vi "getQBData.vi"(8 "error in (no error)":errorcluster, 10 "path":path) -> (0 "error out":errorcluster, 2 "data":string[][](array[string]))   [LabVIEW 2012]
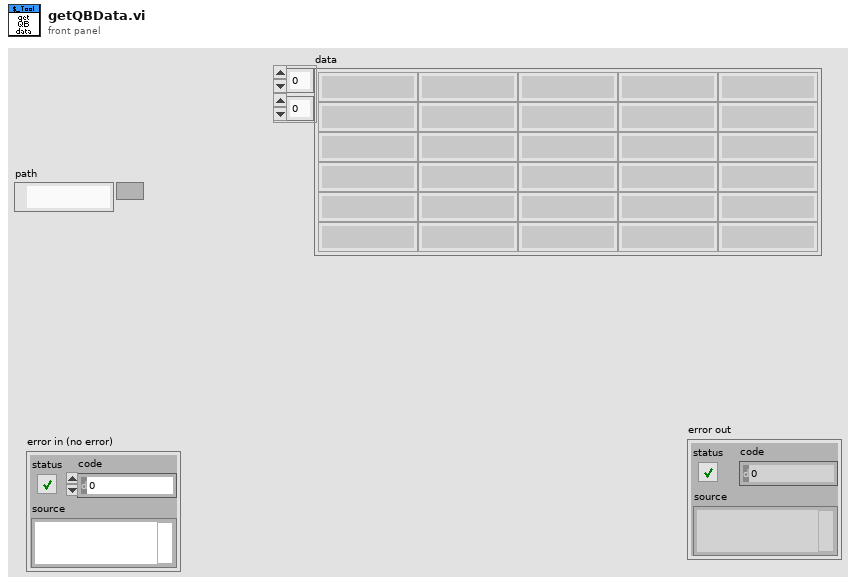
[diagram p1: front panel]
types:
  T1 = cluster{"Excel._Application":refnum<k7>, "Workbooks":refnum<k7>, "Open":refnum<k7>, "Worksheets":refnum<k7>, "Excel._Worksheet":refnum<k7>}
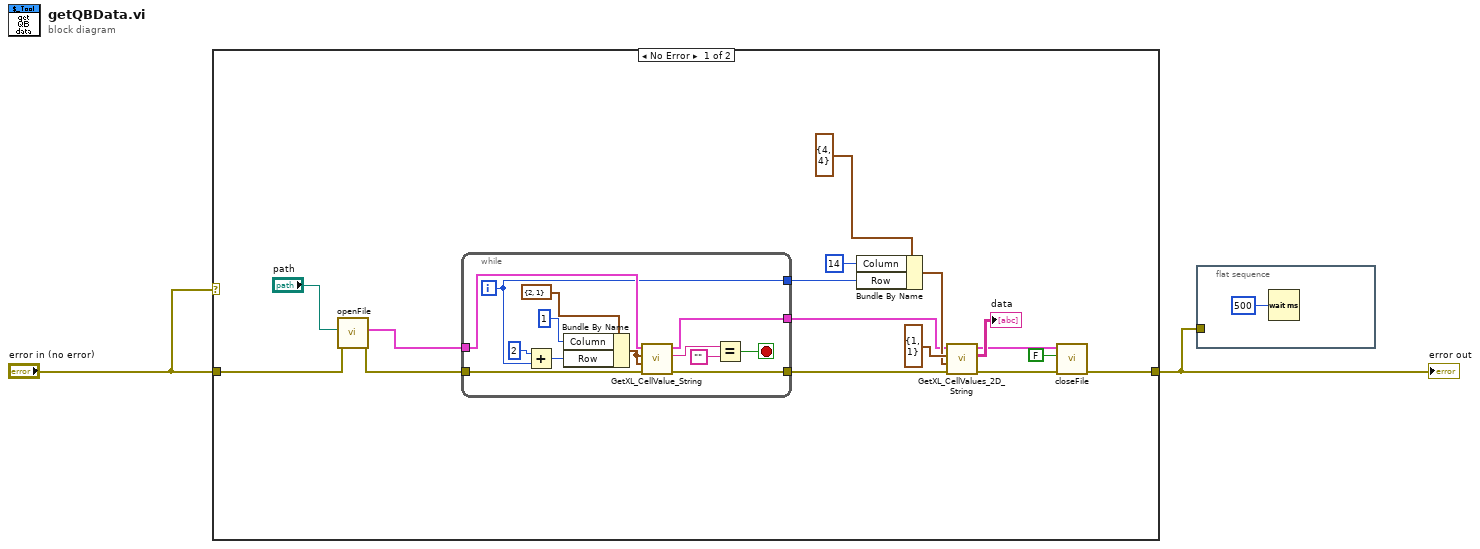
[diagram p0: block diagram]
diagram:
  n1 = case shown="No Error" "error in (no error)" {
    tunnel: "error in (no error)" -> [w8 w32]
    tunnel: [w5 w32] -> w1
    frame No Error {
      n2 = call "openFile.vi"("error in (no error)"=w8, "path"="path") -> ("error out"=w7:errorcluster, "Refnum Cluster Out"=w10:T1)  [unwired: 8 in]
      n3 = while {
        tunnel: w7 -> [w30]
        tunnel: [w29] -> w13
        tunnel: w10 -> [w31]
        tunnel: [w23] -> w15
        tunnel: [w20] -> w12
        i -> [w23]
        stop <- w24 stop-if-true
        n4 = Add(x=2, y=w23) -> (x+y=w22:i32)
        n5 = Bundle By Name(cluster=cluster{"Column":i32, "Row":i32} {"Column"=2, "Row"=1} ("Start"), "Column"=1, "Row"=w22) -> (w19:cluster{"Column":i32, "Row":i32})
        n6 = call <userlib>:"GetXL_CellValue_String.vi"("error in"=w30, "End"=w19, "Start"=w19, "Refnum Cluster In"=w31) -> ("error out"=w29:errorcluster, "data"=w26:string, "Refnum Cluster Out"=w20:T1)  [unwired: 5 in]
        n7 = Equal?(x=w26, y="") -> (x = y?=w24:bool)
      }
      n8 = Bundle By Name(cluster=cluster{"Column":i32, "Row":i32} {"Column"=4, "Row"=4} ("End"), "Column"=14, "Row"=w15) -> (w14:cluster{"Column":i32, "Row":i32})
      n9 = call <userlib>:"GetXL_CellValues_2D_String.vi"("error in"=w13, "End"=w14, "Start"=cluster{"Column":i32, "Row":i32} {"Column"=1, "Row"=1}, "Refnum Cluster In"=w12) -> ("error out"=w6:errorcluster, "data"=→"data":string[][], "Refnum Cluster Out"=w4:T1)  [unwired: 5 in]
      n10 = call "closeFile.vi"("error in (no error)"=w6, "Save? (F)"=FALSE, "Refnum Cluster In"=w4) -> ("error out"=w5:errorcluster)  [unwired: 8 in]
    }
    frame Error {
    }
  }
  "error out" <- w1
  n11 = flat-sequence {
    tunnel: w1 -> [_]
    frame #0 {
      n12 = Wait (ms)(milliseconds to wait=u32 500) -> ()  [unwired: 1 out]
    }
  }
